vi "Keep position above object.vi"(7 "nr of particles":i32, 11 "Position In":T1) -> (0 "Hover":bool, 1 "Roll":dbl format="%#_6f", 2 "Pitch":dbl format="%#_6f", 3 "Position Out":T1)   [LabVIEW 2014]
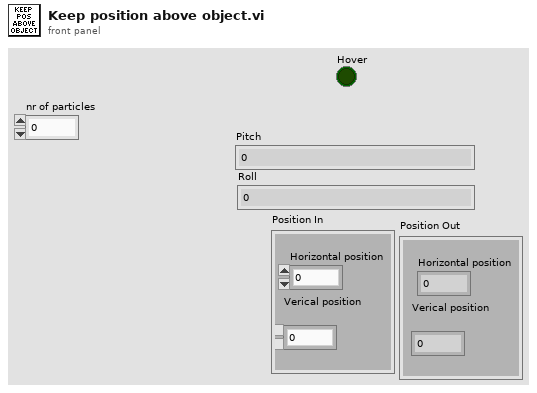
[diagram p1: front panel]
types:
  T1 = cluster{"Horizontal position":dbl, "Verical position\n":dbl}
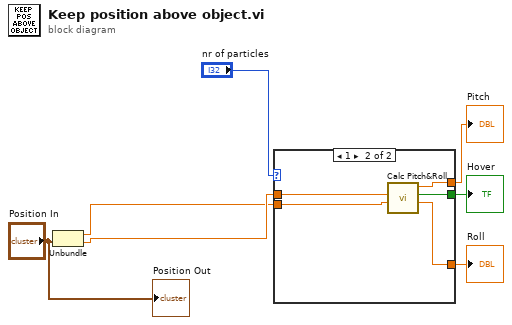
[diagram p0: block diagram]
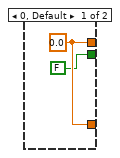
[diagram p2: hidden frame]
diagram:
  n1 = Unbundle("Position In") -> ("Horizontal position"=w2:dbl, "Verical position"=w3:dbl)
  n2 = case shown="1" "nr of particles" {
    tunnel: w3 -> [_ w11]
    tunnel: [w9 w13] -> w7
    tunnel: [FALSE ("Hover") w14] -> w6
    tunnel: [w9 w12] -> w5
    tunnel: w2 -> [_ w10]
    frame 0, Default {
      w9 = 0.0 ("Pitch")
    }
    frame 1 {
      n3 = call "Calc Pitch&Roll.vi"("X"=w10, "Y"=w11) -> ("Roll"=w12:dbl, "Hover"=w14:bool, "Pitch"=w13:dbl)  [unwired: 7 in]
    }
  }
  "Pitch" <- w7
  "Roll" <- w5
  "Hover" <- w6
  "Position Out" <- "Position In"
